vi "Notify_error.vi"(2 "error in":errorcluster, 3 "name":string="ImagingSynch") -> (0 "error out":errorcluster)   [LabVIEW 2010]
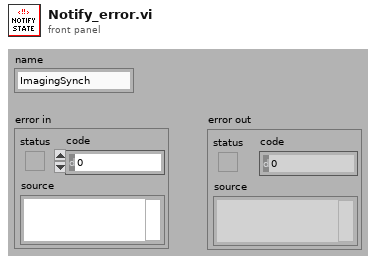
[diagram p1: front panel]
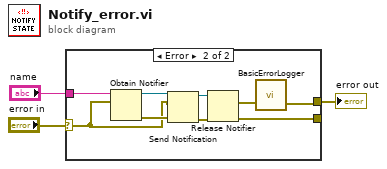
[diagram p0: block diagram]
diagram:
  n1 = case shown="Error" "error in" {
    selector: "error in" -> [_ w7]
    tunnel: [_ w8] -> _
    tunnel: "name" -> [_ w6]
    tunnel: [_ w4] -> w1
    frame No Error {
    }
    frame Error {
      n2 = Obtain Notifier(name (unnamed)=w6, notification data type=w7) -> (notifier out=w12:refnum<notifier>, error out=w11:errorcluster)  [unwired: 2 in, 1 out]
      n3 = Send Notification(notification=w7, notifier=w12, error in (no error)=w11) -> (notifier out=w9:refnum<notifier>, error out=w10:errorcluster)
      n4 = Release Notifier(notifier=w9, error in (no error)=w10) -> (last notification=w5:errorcluster, error out=w8:errorcluster)  [unwired: 1 in, 1 out]
      n5 = call <userlib>:"BasicErrorLogger.vi"("error in"=w5) -> ("error out"=w4:errorcluster)  [unwired: 1 in, 1 out]
    }
  }
  "error out" <- w1
